vi "MHz2uint64.vi"(4 "inMHz":dbl) -> (1 "outu64":u64)   [LabVIEW 2013]
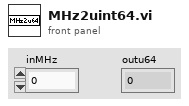
[diagram p1: front panel]
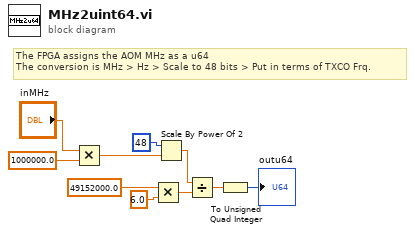
[diagram p0: block diagram]
diagram:
  # "The FPGA assigns the AOM MHz as a u64\nThe conversion is MHz > Hz > Scale to 48 bits > Put in terms of TXCO Frq."
  n1 = Multiply(x="inMHz", y=1000000.0) -> (x*y=w5:dbl)
  n2 = Multiply(x=49152000.0, y=6.0) -> (x*y=w9:dbl)
  n3 = Scale By Power Of 2(n=i16 48, x=w5) -> (x*2^n=w8:dbl)
  n4 = Divide(x=w8, y=w9) -> (x/y=w10:dbl)
  n5 = To Unsigned Quad Integer(1:w10) -> (0:→"outu64":u64)
